vi "resetLabDialog.vi"() -> (3 "T button?":bool)   [LabVIEW 2014]
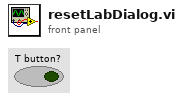
[diagram p1: front panel]
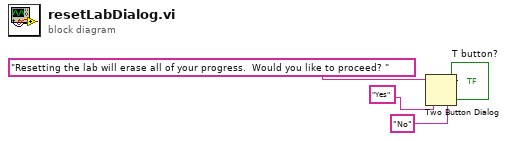
[diagram p0: block diagram]
diagram:
  n1 = Two Button Dialog(message="Resetting the lab will erase all of your progress.  Would you like to proceed? ", 1:"No" ("F button name (\"Cancel\")"), 2:"Yes" ("T button name (\"OK\")")) -> (T button?=→"T button?":bool)
